vi "aal_CIC (complex input) (No State).vi"(7 "aal_CIC (complex input) state in":T1, 8 "Reset":bool, 9 "Stages":i32, 10 "N":i32=1, 11 "x":cdb[](array[numeric])) -> (3 "y":cdb[](array[numeric]), 5 "aal_CIC (complex input) state out":T1)   [LabVIEW 2017, in "NI_AALPro.lvlib"]
uses:
  NI_AALPro.lvlib
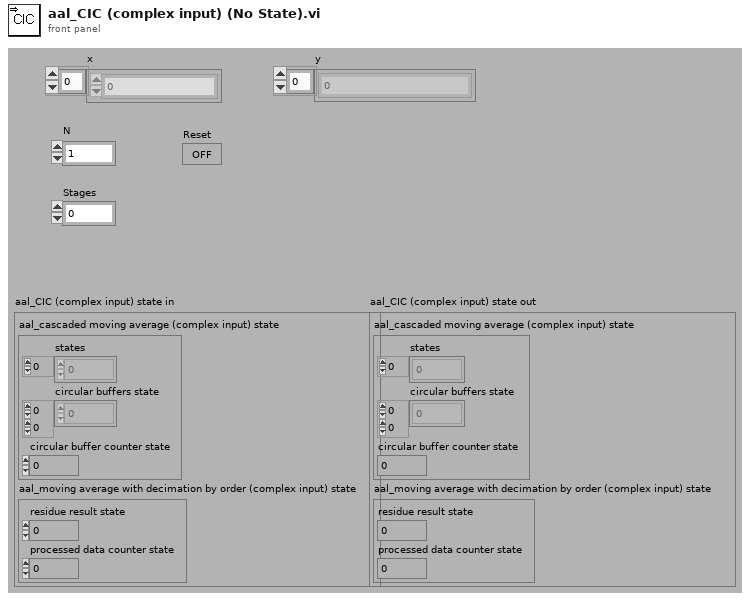
[diagram p1: front panel]
types:
  T1 = cluster{"aal_cascaded moving average (complex input) state":cluster{"states":cdb[], "circular buffers state":cdb[][], "circular buffer counter state":i32}, "aal_moving average with decimation by order (complex input) state":cluster{"residue result state":cdb, "processed data counter state":i32}}
  T2 = cluster{"states":cdb[], "circular buffers state":cdb[][], "circular buffer counter state":i32}
  T3 = cluster{"residue result state":cdb, "processed data counter state":i32}
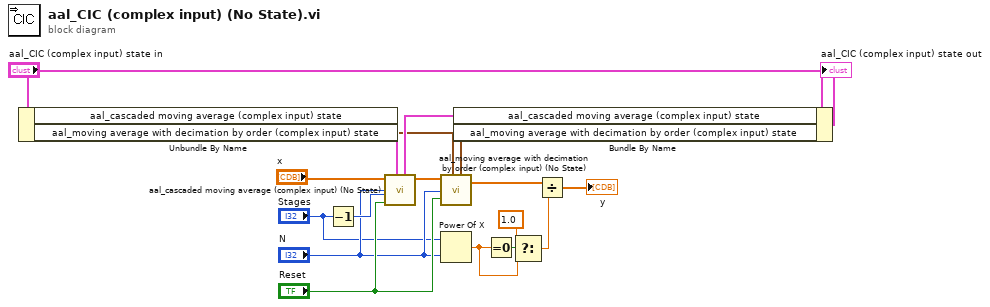
[diagram p0: block diagram]
diagram:
  n1 = Unbundle By Name("aal_CIC (complex input) state in") -> ("aal_cascaded moving average (complex input) state"=w5:T2, "aal_moving average with decimation by order (complex input) state"=w3:T3)
  n2 = Decrement(x="Stages") -> (x-1=w18:i32)
  n3 = call "aal_cascaded moving average (complex input) (No State).vi"("aal_cascaded moving average (complex input) state in"=w5, "Reset"="Reset", "Stages"=w18, "N"="N", "x"="x") -> ("y"=w17:cdb[], "aal_cascaded moving average (complex input) state out"=w4:T2)  [unwired: 5 in]
  n4 = call "aal_moving average with decimation by order (complex input) (No State).vi"("Reset"="Reset", "aal_moving average with decimation by order (complex input) state in"=w3, "N"="N", "x"=w17) -> ("y"=w15:cdb[], "aal_moving average with decimation by order (complex input) state out"=w2:T3)  [unwired: 6 in]
  n5 = Power Of X(1:"N", 2:"Stages") -> (0:w9:dbl)
  n6 = Bundle By Name(cluster="aal_CIC (complex input) state in", "aal_cascaded moving average (complex input) state"=w4, "aal_moving average with decimation by order (complex input) state"=w2) -> (→"aal_CIC (complex input) state out":T1)
  n7 = Equal To 0?(x=w9) -> (x = 0?=w12:bool)
  n8 = Select(t=1.0, s=w12, f=w9) -> (s? t:f=w11:dbl)
  n9 = Divide(x=w15, y=w11) -> (x/y=→"y":cdb[])
